vi "JKISM++ Unregister Status Change.vi"(0 "JKISM Name":string, 5 "Source JKISM Name":string="*", 7 "Status":string, 11 "Error in":errorcluster caption="Error in (no error)") -> (4 "JKISM Name(dup)":string, 15 "Error out":errorcluster)   [LabVIEW 2014, in "JKI State Machine++.lvlib"]
doc: "Unregister the notification of other JKISM++ Module's status change.\n\n<b>Inputs:</b>\n - <b>JKISM Name</b>: JKISM Module name.\n - <b>Source JKISM Name</b>: JKISM who generates the status. You can use '*' for all modules generated the same <b>Status</b>\n - <b>Status</b>: The status string\n - <b>Error in</b>: Error cluster\n\n<b>Outputs:</b>\n - <b>JKISM Name(dup)</b>: return <b>JKISM Name</b>\n - <b>Error out</b>: Error cluster"
uses:
  JKI State Machine++.lvlib
  _Support/FGV-BroadcastRegistry/Operation-BroadcastRegistry.ctl
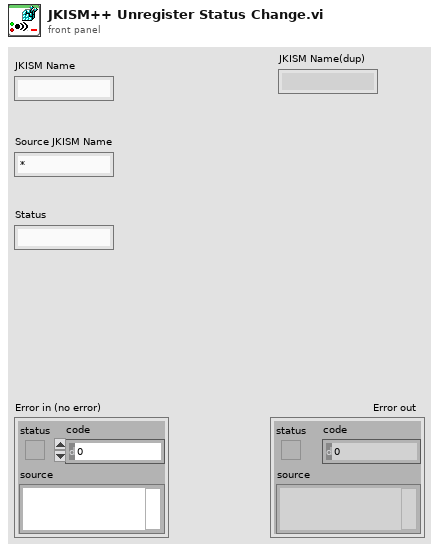
[diagram p1: front panel]
types:
  T1 = typedef "JKI State Machine++.lvlib/Operation-BroadcastRegistry.ctl" = enum16{"Delete Source Module", "Delete Target Module", "Remove Module", "Register", "Unregister", "Check"}
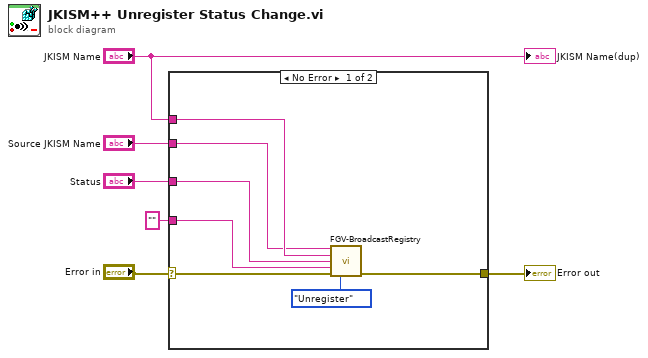
[diagram p0: block diagram]
diagram:
  n1 = case shown="No Error" "Error in" {
    selector: "Error in" -> [w12 w14]
    tunnel: [w11 w14] -> w5
    tunnel: "" ("Response Message") -> [w10 _]
    tunnel: "Status" -> [w9 _]
    tunnel: "Source JKISM Name" -> [w7 _]
    tunnel: "JKISM Name" -> [w8 _]
    frame No Error {
      n2 = call "FGV-BroadcastRegistry.vi"("Source"=w7, "Target"=w8, "Message"=w9, "Response Message In"=w10, "Error in"=w12, "Operation"=Operation-BroadcastRegistry."Unregister") -> ("Error out"=w11:errorcluster)  [unwired: 7 in, 2 out]
    }
    frame Error {
    }
  }
  "Error out" <- w5
  "JKISM Name(dup)" <- "JKISM Name"
